vi "StringManipulation.vi"(0 "Input String":string, 5 "Stop":bool) -> ()   [LabVIEW 2020]
panel:
  # "String Manipulation and Event Handling"
  # "Description:\n1. When the input is given the case will be changed.\n2. While closing the vi a dialogue will pop up wheather to close\nthe vi or not. If not it will stop the running of VI"
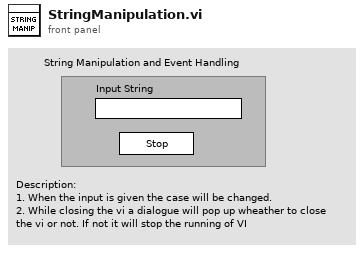
[diagram p1: front panel]
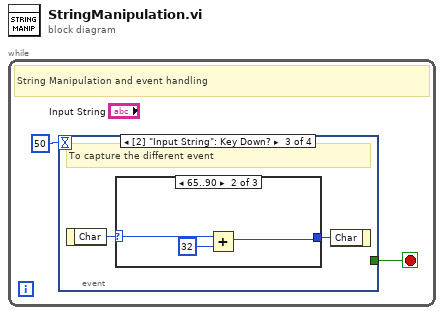
[diagram p0: block diagram]
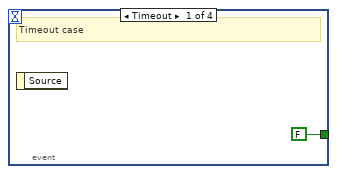
[diagram p2: hidden frame]
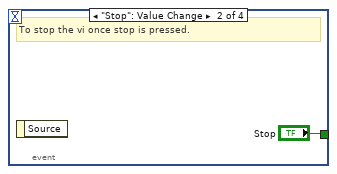
[diagram p3: hidden frame]
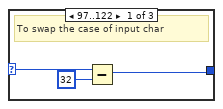
[diagram p4: hidden frame]
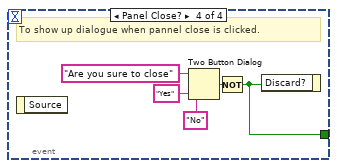
[diagram p6: hidden frame]
diagram:
  n1 = while {
    stop <- w2 stop-if-true
    # "String Manipulation and event handling"
    n2 = event shown="[2] \"Input String\": Key Down?" {
      selector: _ -> [_ _ _ _]
      dyn-events: _ -> [_ _ _ _]
      timeout: 50 -> [_ _ _ _]
      tunnel: [FALSE "Stop" _ w14] -> w2
      event Timeout {
        # "Timeout case"
        n3 = event-data() -> ()  [unwired: 1 in, 1 out]
      }
      event "Stop": Value Change {
        # "To stop the vi once stop is pressed."
        n4 = event-data() -> ()  [unwired: 1 in, 1 out]
      }
      event "Input String": Key Down? {
        # "To capture the different event"
        n5 = event-data() -> ("Char"=w6:i16)  [unwired: 1 in]
        n6 = case shown="65..90" w6 {
          selector: w6 -> [w9 w12 w13]
          tunnel: [w7 w10 w13] -> w5
          frame 97..122 {
            # "To swap the case of input char"
            n7 = Subtract(x=w9, y=i16 32) -> (x-y=w7:i16)
          }
          frame 65..90 {
            n8 = Add(x=w12, y=i16 32) -> (x+y=w10:i16)
          }
          frame Default {
          }
        }
        n9 = event-data("Char"=w5) -> ()  [unwired: 1 in, 1 out]
      }
      event Panel Close? {
        # "To show up dialogue when pannel close is clicked."
        n10 = event-data() -> ()  [unwired: 1 in, 1 out]
        n11 = Two Button Dialog(message="Are you sure to close", 1:"No" ("F button name (\"Cancel\")"), 2:"Yes" ("T button name (\"OK\")")) -> (T button?=w15:bool)
        n12 = Not(x=w15) -> (.not. x?=w14:bool)
        n13 = event-data("Discard?"=w14) -> ()  [unwired: 1 in, 1 out]
      }
    }
  }
